vi "SUB-BLE Rx Wait.vi"(5 "Timeout(ms)":u16) -> (2 "RxReady":bool=TRUE)   [LabVIEW 2015]
doc: "Use this template to create an application that executes repeatedly until you click the Stop button. This template polls the state of the Stop button and does not use events. Use the Top-Level Application template (not available in the Base package) to create a single-loop application with event handling."
uses:
  Global 1.vi
panel:
  out "BLE Packet (buf)":u8[](array[numeric])
  out "BLE Packet (data)":u8[](array[numeric])
  out "BLE Packet":bool=TRUE
  # "BLE 데이터 수신 대기"
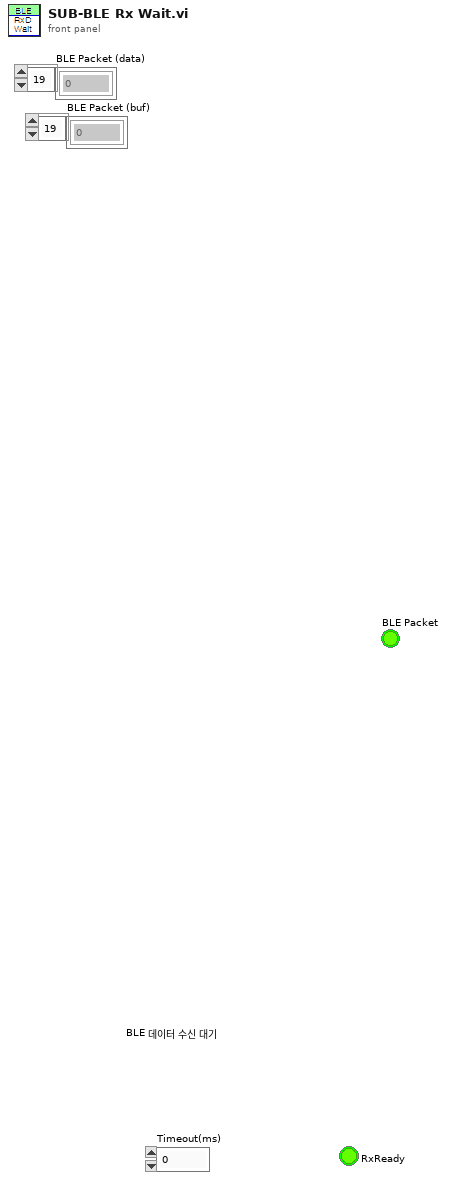
[diagram p1: front panel]
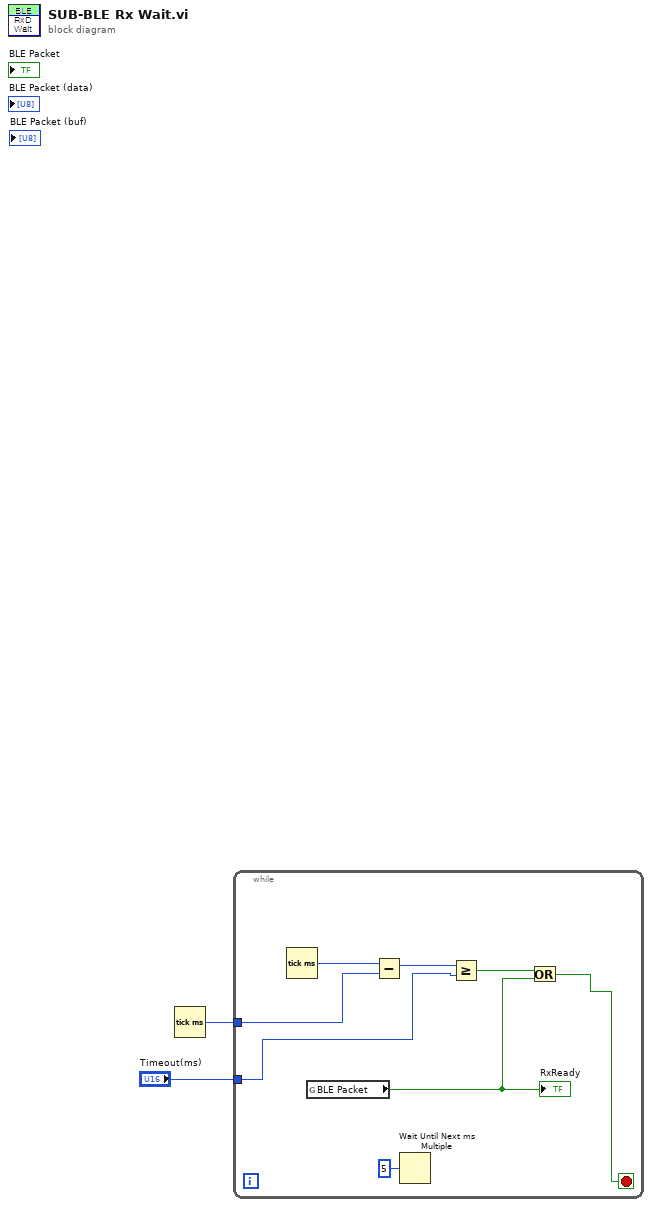
[diagram p0: block diagram]
diagram:
  n1 = Tick Count (ms)() -> (millisecond timer value=w2:u32)
  n2 = while {
    tunnel: w2 -> [w8]
    tunnel: "Timeout(ms)" -> [w4]
    stop <- w7 stop-if-true
    n3 = Tick Count (ms)() -> (millisecond timer value=w9:u32)
    n4 = global read "Global 1.vi" "BLE Packet"() -> (w6:bool)
    "RxReady" <- w6
    n5 = Subtract(x=w9, y=w8) -> (x-y=w5:u32)
    n6 = Wait Until Next ms Multiple(millisecond multiple=u32 5 ("ms 배수")) -> ()  [unwired: 1 out]
    n7 = Greater Or Equal?(x=w5, y=w4) -> (x >= y?=w3:bool)
    n8 = Or(x=w3, y=w6) -> (x .or. y?=w7:bool)
  }
